vi "ReadConfigFile.vi"(8 "ErrorIn":errorcluster, 11 "ClusterIn":T1={"MainQ"=refnum, "User"={"Lvl"=enum."Admin", "Pwd"=""}, "Stat"={"SysState"=enum."Init"}, "Paths"={"CfgFile"=path "", "LogFolder"=path "", "LogFile"=path ""}, "HW"={"HW?"=FALSE, "HWMode"=enum."RTHW_Init", "Refs"={"Visa"="GPIB0::2::INSTR"}}, "RTConfig"={"Arm"=FALSE, "Number"=0.0, "String"=""}}) -> (0 "ErrorOut":errorcluster, 3 "ClusterOut":T1={"MainQ"=refnum, "User"={"Lvl"=enum."Admin", "Pwd"=""}, "Stat"={"SysState"=enum."Init"}, "Paths"={"CfgFile"=path "", "LogFolder"=path "", "LogFile"=path ""}, "HW"={"HW?"=FALSE, "HWMode"=enum."RTHW_Init", "Refs"={"Visa"="GPIB0::2::INSTR"}}, "RTConfig"={"Arm"=FALSE, "Number"=0.0, "String"=""}})   [LabVIEW 2018]
doc: "Attempt to read the configuration (INI) file specified in ClusterIn.Paths.CfgFile. If the file exists, the INI file is read and elements are filled in to the cluster. If it does not exist, a new INI file is created using default values.\n\nAdd elements to this VI for each cluster element that you wish to reload.\n\nCopyright © 2011 Epimedia, Inc. All Rights Reserved.\n\nThe Epimedia Application Library is Copyright © 2009-2011 Epimedia, Inc. \nAll Rights Reserved. Used under license."
uses:
  Controls/MasterCluster_RT.ctl
  Queue/RTMainQueueElements.ctl
  Controls/UserCluster_RT.ctl
  Controls/UserLevelEnum_RT.ctl
  Controls/SystemStatusCluster_RT.ctl
  Controls/SystemStateEnum_RT.ctl
  Controls/PathsCluster_RT.ctl
  Controls/HWCluster_RT.ctl
  Queue/HWQueueElements.ctl
  Controls/HWRefsCluster_RT.ctl
  Controls/RT_Config.ctl
  <vilib>/Utility/config.llb/Read Key (Boolean).vi
  <vilib>/Utility/config.llb/Read Key (Double).vi
  <vilib>/Utility/config.llb/Read Key (String).vi
  <vilib>/Utility/config.llb/NI_LVConfig.lvlib
panel:
  # "Copyright © 2011 Epimedia, Inc. All Rights Reserved.\n\nThe Epimedia Application Library is Copyright © 2009-2011 Epimedia, Inc. \nAll Rights Reserved. Used under license."
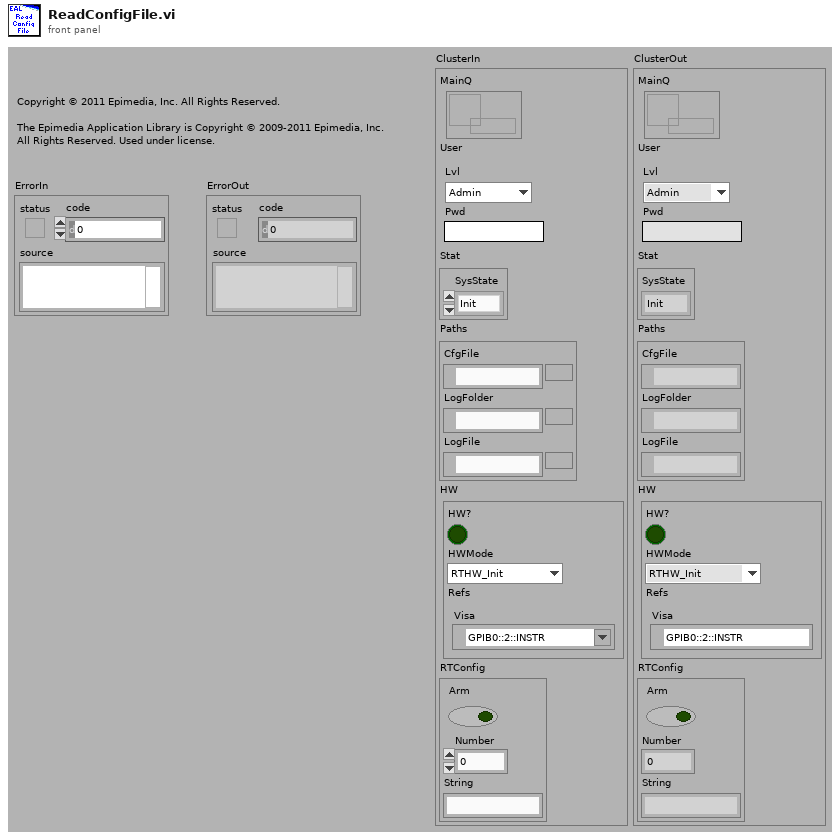
[diagram p1: front panel]
types:
  T1 = typedef "MasterCluster_RT.ctl" = cluster{"MainQ":refnum<queue>, "User":T2, "Stat":T4, "Paths":T6, "HW":T7, "RTConfig":T10}
  T2 = typedef "UserCluster_RT.ctl" = cluster{"Lvl":T3, "Pwd":string}
  T3 = typedef "UserLevelEnum_RT.ctl" = enum16{"Admin", "Operator"}
  T4 = typedef "SystemStatusCluster_RT.ctl" = cluster{"SysState":T5}
  T5 = typedef "SystemStateEnum_RT.ctl" = enum16{"Init", "Idle", "Running", "Error", "Exit"}
  T6 = typedef "PathsCluster_RT.ctl" = cluster{"CfgFile":path, "LogFolder":path, "LogFile":path}
  T7 = typedef "HWCluster_RT.ctl" = cluster{"HW?":bool, "HWMode":T8, "Refs":T9}
  T8 = typedef "HWQueueElements.ctl" = enum16{"RTHW_Init", "RTHW_UpdtCfg", "RTHW_Start", "RTHW_Pause", "RTHW_Run", "RTHW_Cls", "RTHW_Exit"}
  T9 = typedef "HWRefsCluster_RT.ctl" = cluster{"Visa":refnum<visa-resource-name>}
  T10 = typedef "RT_Config.ctl" = cluster{"Arm":bool, "Number":dbl, "String":string}
  T11 = typedef "NI_LVConfig.lvlib/Config Data RefNum.ctl" = refnum<k1>
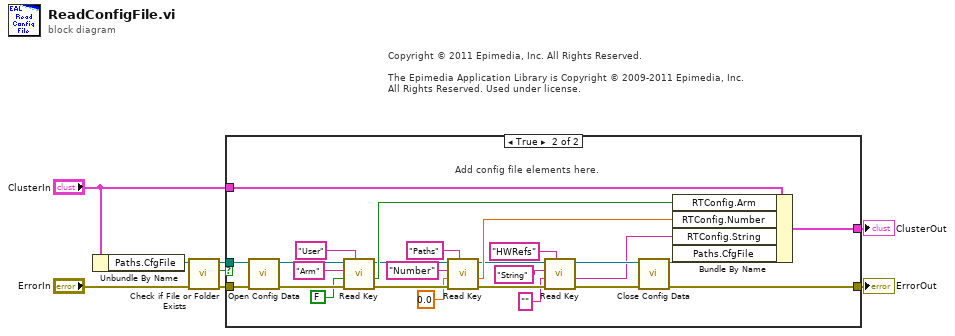
[diagram p0: block diagram]
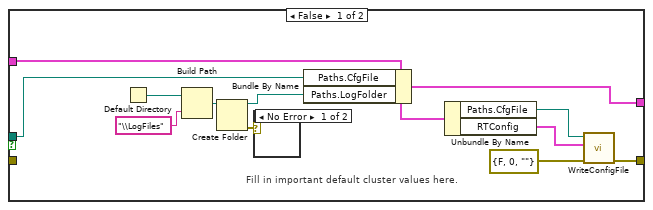
[diagram p2: hidden frame]
diagram:
  # "Copyright © 2011 Epimedia, Inc. All Rights Reserved.\n\nThe Epimedia Application Library is Copyright © 2009-2011 Epimedia, Inc. \nAll Rights Reserved. Used under license."
  n1 = Unbundle By Name("ClusterIn") -> ("Paths.CfgFile"=w5:path)
  n2 = call <vilib>:"Check if File or Folder Exists.vi"("error in (no error)"="ErrorIn", "path"=w5) -> ("error out"=w1:errorcluster, "file or folder exists?"=w2:bool, "dup path"=w4:path)  [unwired: 7 out]
  n3 = case shown="True" w2 {
    tunnel: [w20 w46] -> w8
    tunnel: [w19 w44] -> w7
    tunnel: w4 -> [w17 w42]
    tunnel: "ClusterIn" -> [w11 w41]
    tunnel: w1 -> [_ w40]
    frame False {
      # "Fill in important default cluster values here."
      n4 = Default Directory() -> (w12:path)
      n5 = Build Path(base path=w12, name or relative path="\\LogFiles") -> (appended path=w14:path)
      n6 = Create Folder(path (use dialog)=w14) -> (created path=w13:path, error out=w15:errorcluster)  [unwired: 2 in, 1 out]
      n7 = case shown="No Error" w15 {
        frame No Error {
        }
        frame Error {
        }
      }
      n8 = Bundle By Name(cluster=w11, "Paths.CfgFile"=w17, "Paths.LogFolder"=w13) -> (w19:T1)
      n9 = Unbundle By Name(w11) -> ("Paths.CfgFile"=w9:path, "RTConfig"=w10:T10)
      n10 = call "WriteConfigFile.vi"("ErrorIn"=errorcluster {"status"=FALSE, "code"=0, "source"=""}, "RTConfig"=w10, "configuration file path"=w9) -> ("ErrorOut"=w20:errorcluster)  [unwired: 8 out]
    }
    frame True {
      # "Add config file elements here."
      n11 = call <vilib>:"Open Config Data.vi"("error in (no error)"=w40, "configuration file path"=w42) -> ("error out"=w36:errorcluster, "refnum"=w35:T11)  [unwired: 7 in, 1 out]
      n12 = call-poly <vilib>:"Read Key.vi"("section"="User" ("key"), "error in (no error)"=w36, "default value"=FALSE, "key"="Arm", "refnum"=w35) -> ("error out"=w30:errorcluster, "value"=w39:bool, "refnum out"=w31:T11)  [unwired: 4 out]
      n13 = call-poly <vilib>:"Read Key.vi"("section"="Paths" ("key"), "error in (no error)"=w30, "default value"=0.0, "key"="Number", "refnum"=w31) -> ("error out"=w29:errorcluster, "value"=w33:dbl, "refnum out"=w28:T11)  [unwired: 4 out]
      n14 = call-poly <vilib>:"Read Key.vi"("section"="HWRefs" ("key"), "error in (no error)"=w29, "default value"="", "key"="String", "refnum"=w28) -> ("error out"=w27:errorcluster, "value"=w26:string, "refnum out"=w32:T11)  [unwired: 1 in, 3 out]
      n15 = call <vilib>:"Close Config Data.vi"("error in (no error)"=w27, "refnum"=w32) -> ("error out"=w46:errorcluster, "file path"=w45:path)  [unwired: 1 in, 7 out]
      n16 = Bundle By Name(cluster=w41, "RTConfig.Arm"=w39, "RTConfig.Number"=w33, "RTConfig.String"=w26, "Paths.CfgFile"=w45) -> (w44:T1)
    }
  }
  "ErrorOut" <- w8
  "ClusterOut" <- w7
